vi "Get Cursor Position.vi"(8 "Error In":errorcluster, 11 "Graph Ref In":refnum<vi>) -> (0 "Error Out":errorcluster, 2 "# of Samples":i32, 3 "Graph Ref Out":refnum<vi>)   [LabVIEW 2019, in "Graph Tools.lvlib"]
doc: "Get Graph Cursor Position."
uses:
  Graph Tools.lvlib
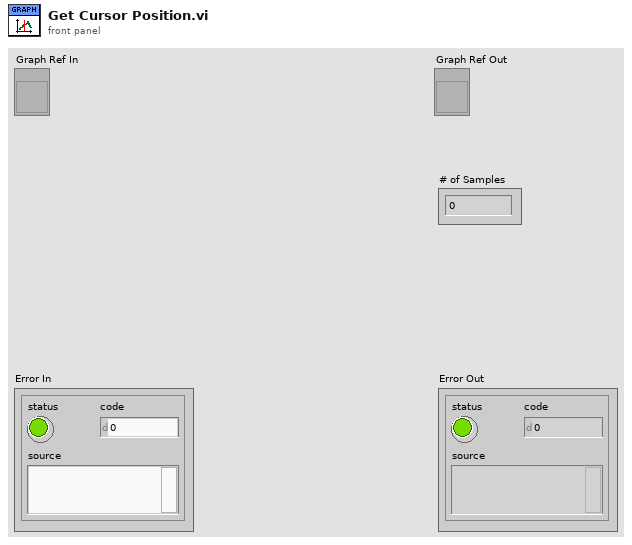
[diagram p1: front panel]
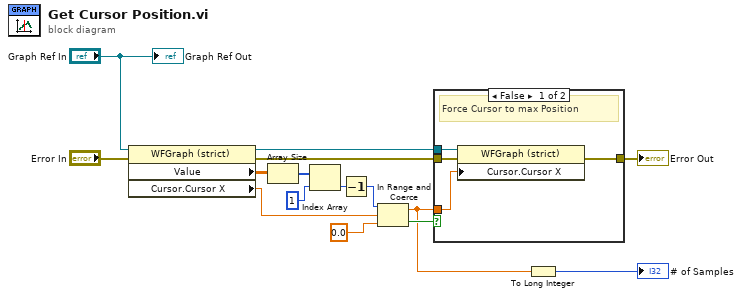
[diagram p0: block diagram]
diagram:
  n1 = property on="Property Node" class="WFGraph (strict)"(reference="Graph Ref In", error in="Error In") -> (reference out=w13:refnum<vi>, error out=w3:errorcluster, "Value"=w10:dbl[][], "Cursor.Cursor X"=w15:dbl)
  n2 = Array Size(array=w10) -> (size(s)=w9:i32[])
  n3 = Index Array(array=w9, index=1) -> (element=w7:i32)
  n4 = Decrement(x=w7) -> (x-1=w6:i32)
  n5 = In Range and Coerce(upper limit=w6, x=w15, lower limit=0.0) -> (coerced(x)=w11:dbl, In Range?=w12:bool)
  n6 = case shown="False" w12 {
    tunnel: w13 -> [w19 _]
    tunnel: w11 -> [w18 _]
    tunnel: w3 -> [w17 w20]
    tunnel: [w16 w20] -> w2
    frame False {
      # "Force Cursor to max Position"
      n7 = property on="Property Node" class="WFGraph (strict)"(reference=w19, error in=w17, "Cursor.Cursor X"=w18) -> (error out=w16:errorcluster)  [unwired: 1 out]
    }
    frame True {
    }
  }
  "Error Out" <- w2
  n8 = To Long Integer(number=w11) -> (32bit integer=→"# of Samples":i32)
  "Graph Ref Out" <- "Graph Ref In"
